vi "Rachel_Wheel_Test.vi"() -> ()   [LabVIEW 2017]
uses:
  <vilib>/myRIO/Instrument Drivers/Onboard IO/PWM/typedefs/PWM Reference.ctl
  <vilib>/myRIO/Common/Instrument Driver Framework/Utilities/typedefs/myRIO Generic Hardware Reference.ctl
  <vilib>/myRIO/Common/Instrument Driver Framework/Utilities/typedefs/Hardware Version Enum.ctl
  <vilib>/myRIO/Common/Instrument Driver Framework/Utilities/typedefs/myRIO v1.0 Reference.ctl
  <vilib>/myRIO/Common/Instrument Driver Framework/Utilities/typedefs/Generic FPGA Reference.ctl
  <vilib>/myRIO/Common/Instrument Driver Framework/myRIO v1.0/PWM/typedefs/PWM Channels Enum.ctl
  <vilib>/myRIO/Instrument Drivers/Onboard IO/PWM/typedefs/PWM Configuration.ctl
  <vilib>/userdefined/High Color/nirio_resource_hc.ctl
  <vilib>/myRIO/Common/Instrument Driver Framework/Utilities/vis/Is FPGA Ref Available.vi
  <vilib>/myRIO/Common/Instrument Driver Framework/myRIO v1.0/PWM/vis/myRIO v1.1 Open PWM.vi
  <vilib>/myRIO/Instrument Drivers/Onboard IO/PWM/vis/Set Duty Cycle and Frequency.vi
  <vilib>/myRIO/Common/Instrument Driver Framework/Utilities/vis/Validate Channels.vi
  <vilib>/myRIO/Common/Instrument Driver Framework/myRIO v1.0/PWM/vis/myRIO v1.0 Reserve PWM.vi
  <vilib>/myRIO/Common/Instrument Driver Framework/myRIO v1.0/PWM/vis/myRIO v1.0 Build MUX Configuration PWM.vi
  <vilib>/myRIO/Common/Instrument Driver Framework/myRIO v1.0/Resource Manager/vis/myRIO v1.0 Reserve Channel List.vi
  <vilib>/myRIO/Common/Instrument Driver Framework/myRIO v1.0/Resource Manager/vis/myRIO v1.0 Create Configuration List.vi
  <vilib>/myRIO/Common/Instrument Driver Framework/myRIO v1.0/Resource Manager/vis/myRIO v1.0 Reserve Channel.vi
  <vilib>/myRIO/Common/Instrument Driver Framework/myRIO v1.0/Resource Manager/vis/myRIO v1.0 Unreserve Channel.vi
  <vilib>/myRIO/Common/Instrument Driver Framework/myRIO v1.0/Resource Manager/vis/myRIO v1.0 Build Mutex Name.vi
  <vilib>/Utility/VariantDataType/GetNumericInfo.vi
  <vilib>/Utility/error.llb/Error Cluster From Error Code.vi
  <vilib>/myRIO/Common/Instrument Driver Framework/myRIO v1.0/myRIO v1.1 Open.vi
  <vilib>/myRIO/Common/Instrument Driver Framework/Utilities/vis/IO Manager.vi
  <vilib>/myRIO/Common/Instrument Driver Framework/Utilities/vis/Configuration Manager.vi
  <vilib>/myRIO/Common/Instrument Driver Framework/myRIO v1.0/Resource Manager/vis/myRIO v1.0 Configure IO.vi
  <vilib>/myRIO/Common/Instrument Driver Framework/myRIO v1.0/myRIO v1.0 Close.vi
  <vilib>/myRIO/Common/Instrument Driver Framework/myRIO v1.0/PWM/vis/myRIO v1.0 Write PWM.vi
  <vilib>/myRIO/Express VI/Onboard IO/PWM/PWM Express VI.xnode
  <vilib>/myRIO/Instrument Drivers/Onboard IO/PWM/vis/myRIO PWM Open.xnode
  <vilib>/myRIO/Instrument Drivers/Onboard IO/PWM/PWM.lvlib
panel:
  out "x*y 3":dbl
  out "x*y 2":dbl
  out "x*y":dbl
  out "O3":dbl
  out "O2":dbl
  out "O1":dbl
  in  "Max Speed":dbl
  in  "Heading Bias":dbl
  in  "1/R":dbl
  in  "L":dbl
  in  "Y":dbl
  in  "X":dbl
  in  "Boolean":bool
  in  "Slide 3":dbl(slide) scale=0.065..0.085
  in  "Slide 2":dbl(slide) scale=0.065..0.085
  in  "Slide":dbl(slide) scale=0.065..0.085
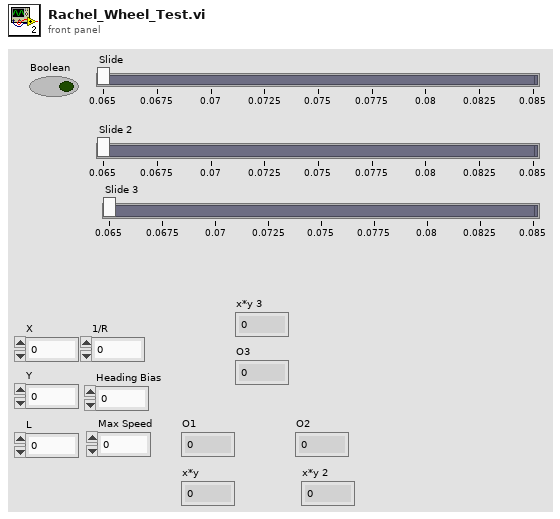
[diagram p1: front panel]
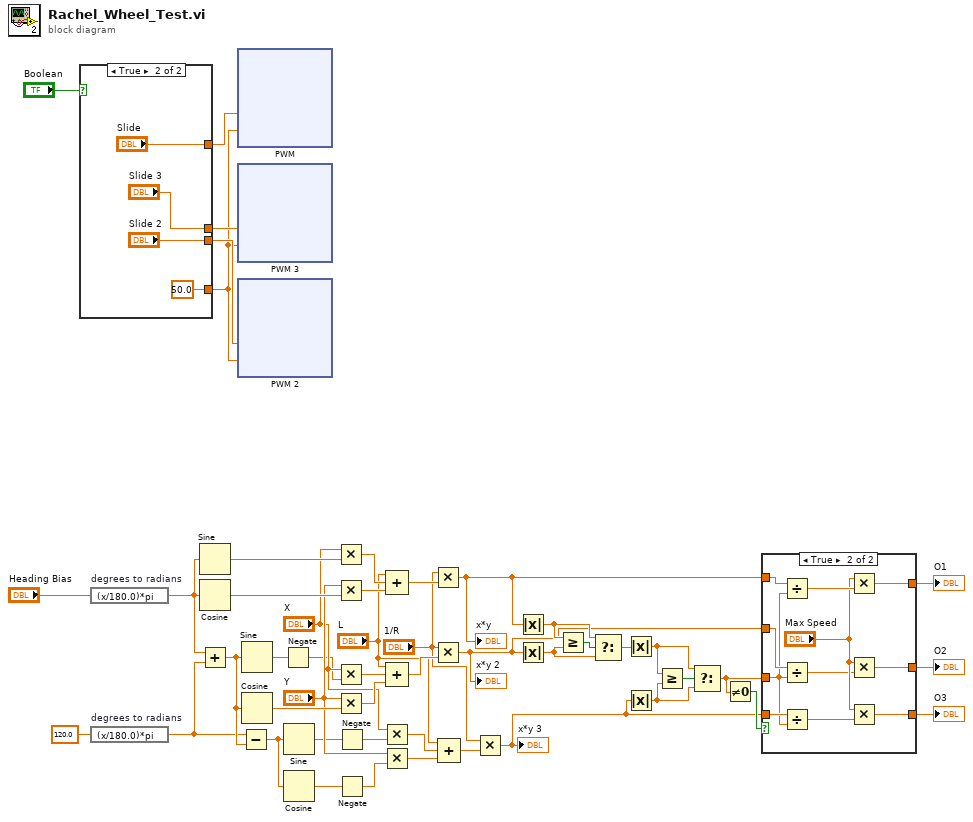
[diagram p0: block diagram]
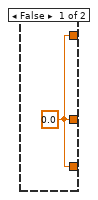
[diagram p2: hidden frame]
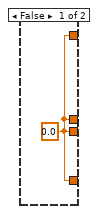
[diagram p3: hidden frame]
diagram:
  n1 = case shown="True" "Boolean" {
    tunnel: [w49 "Slide"] -> w48
    tunnel: [w49 "Slide 2"] -> w47
    tunnel: [w49 "Slide 3"] -> w46
    tunnel: [w49 50.0] -> w45
    frame False {
      w49 = 0.0
    }
    frame True {
    }
  }
  n2 = expression code="(x/180.0)*pi" "degrees to radians"("Heading Bias") -> (w3:dbl)
  n3 = expression code="(x/180.0)*pi" "degrees to radians"(120.0 ("y")) -> (w1:dbl)
  n4 = Sine(x=w3) -> (sin(x)=w43:dbl)
  n5 = Cosine(x=w3) -> (cos(x)=w42:dbl)
  n6 = Add(x=w3, y=w1) -> (x+y=w8:dbl)
  n7 = xnode "PWM"("Duty Cycle"=w48, "Frequency [Hz]"=w45) -> ()  [unwired: 1 in, 1 out]
  n8 = xnode "PWM 3"("Duty Cycle"=w46, "Frequency [Hz]"=w45) -> ()  [unwired: 1 in, 1 out]
  n9 = xnode "PWM 2"("Duty Cycle"=w47, "Frequency [Hz]"=w45) -> ()  [unwired: 1 in, 1 out]
  n10 = Subtract(x=w1, y=w8) -> (x-y=w9:dbl)
  n11 = Sine(x=w8) -> (sin(x)=w11:dbl)
  n12 = Cosine(x=w8) -> (cos(x)=w38:dbl)
  n13 = Negate(x=w11) -> (-x=w10:dbl)
  n14 = Sine(x=w9) -> (sin(x)=w13:dbl)
  n15 = Cosine(x=w9) -> (cos(x)=w15:dbl)
  n16 = Multiply(x="X", y=w43) -> (x*y=w41:dbl)
  n17 = Multiply(x="Y", y=w42) -> (x*y=w40:dbl)
  n18 = Multiply(x="X", y=w10) -> (x*y=w37:dbl)
  n19 = Multiply(x="Y", y=w38) -> (x*y=w36:dbl)
  n20 = Negate(x=w13) -> (-x=w12:dbl)
  n21 = Negate(x=w15) -> (-x=w14:dbl)
  n22 = Multiply(x="X", y=w12) -> (x*y=w34:dbl)
  n23 = Multiply(x="Y", y=w14) -> (x*y=w33:dbl)
  n24 = Compound Arithmetic op=ADD("L", w41, w40) -> (w39:dbl)
  n25 = Compound Arithmetic op=ADD("L", w37, w36) -> (w35:dbl)
  n26 = Multiply(x="1/R", y=w39) -> (x*y=w17:dbl)
  "x*y" <- w17
  n27 = Multiply(x="1/R", y=w35) -> (x*y=w18:dbl)
  "x*y 2" <- w18
  n28 = Compound Arithmetic op=ADD("L", w34, w33) -> (w32:dbl)
  n29 = Multiply(x="1/R", y=w32) -> (x*y=w19:dbl)
  "x*y 3" <- w19
  n30 = Absolute Value(x=w17) -> (abs(x)=w27:dbl)
  n31 = Absolute Value(x=w18) -> (abs(x)=w26:dbl)
  n32 = Greater Or Equal?(x=w27, y=w26) -> (x >= y?=w25:bool)
  n33 = Select(t=w27, s=w25, f=w26) -> (s? t:f=w21:dbl)
  n34 = Absolute Value(x=w21) -> (abs(x)=w24:dbl)
  n35 = Absolute Value(x=w19) -> (abs(x)=w23:dbl)
  n36 = Greater Or Equal?(x=w24, y=w23) -> (x >= y?=w22:bool)
  n37 = Select(t=w24, s=w22, f=w23) -> (s? t:f=w16:dbl)
  n38 = Not Equal To 0?(x=w16) -> (x != 0?=w20:bool)
  n39 = case shown="True" w20 {
    tunnel: w19 -> [_ w65]
    tunnel: w18 -> [_ w64]
    tunnel: w17 -> [_ w63]
    tunnel: w16 -> [_ w62]
    tunnel: [w54 w57] -> w7
    tunnel: [w54 w56] -> w6
    tunnel: [w54 w55] -> w5
    frame False {
      w54 = 0.0
    }
    frame True {
      n40 = Divide(x=w63, y=w62) -> (x/y=w61:dbl)
      n41 = Divide(x=w64, y=w62) -> (x/y=w58:dbl)
      n42 = Divide(x=w65, y=w62) -> (x/y=w59:dbl)
      n43 = Multiply(x="Max Speed", y=w61) -> (x*y=w55:dbl)
      n44 = Multiply(x="Max Speed", y=w58) -> (x*y=w56:dbl)
      n45 = Multiply(x="Max Speed", y=w59) -> (x*y=w57:dbl)
    }
  }
  "O1" <- w5
  "O2" <- w6
  "O3" <- w7
